vi "getTemperatures (SubVI).vi"(8 "error in (no error)":errorcluster, 10 "file path (dialog if empty)":path, 11 "Application in":refnum<vi>) -> (0 "error out":errorcluster, 1 "Application ref out":refnum<vi>, 2 "TCryo":dbl, 3 "TSTM":dbl)   [LabVIEW 2014]
uses:
  <vilib>/Utility/file.llb/Write To Spreadsheet File (DBL).vi
  <vilib>/Utility/file.llb/Read From Spreadsheet File (DBL).vi
  <userlib>/Nanonis Prog Interface V5/Nanonis Prog Interface.lvlib
  <vilib>/gmath/NI_Gmath.lvlib
panel:
  out "error":i32
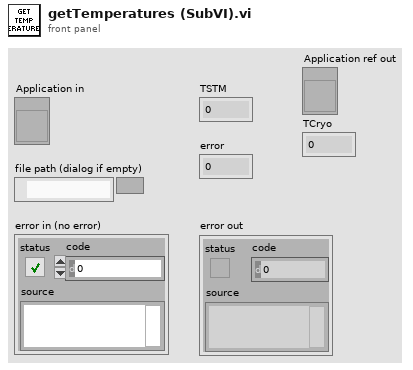
[diagram p1: front panel]
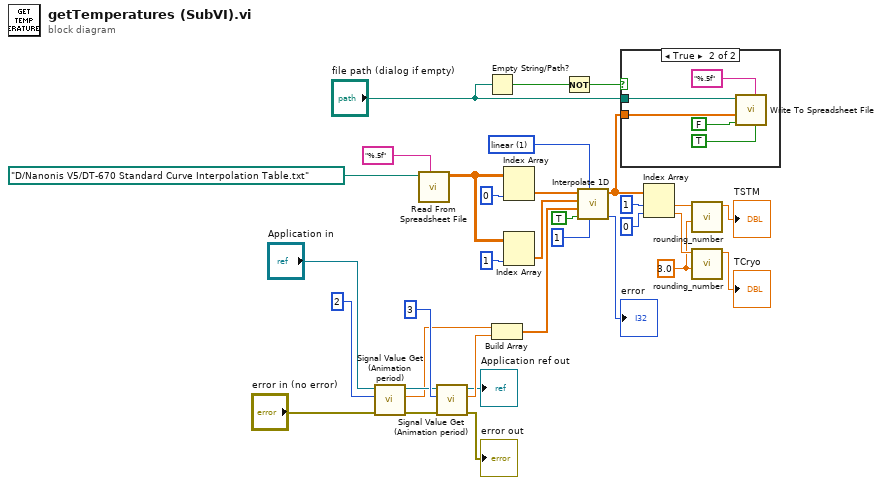
[diagram p0: block diagram]
diagram:
  w1 = 3.0 ("decimal Places")
  w21 = 1 items=["nearest", "linear", "spline", "cubic Hermite", "Lagrange"] ("method")
  n1 = call <userlib>:"Signal Value Get (Animation period).vi"("error in (no error)"="error in (no error)", "Signal index (0-47)"=i8 2, "Application ref in"="Application in") -> ("error out"=w30:errorcluster, "Signal value"=w24:sgl, "Application ref out"=w31:refnum<vi>)  [unwired: 5 in]
  n2 = call-poly <vilib>:"Read From Spreadsheet File.vi"("format (%.3f)"="%.5f", "file path (dialog if empty)"=path "D:/Nanonis V5/DT-670 Standard Curve Interpolation Table.txt") -> ("all rows"=w18:dbl[][])  [unwired: 5 in, 4 out]
  n3 = call <userlib>:"Signal Value Get (Animation period).vi"("error in (no error)"=w30, "Signal index (0-47)"=i8 3, "Application ref in"=w31) -> ("error out"=→"error out":errorcluster, "Signal value"=w32:sgl, "Application ref out"=→"Application ref out":refnum<vi>)  [unwired: 5 in]
  n4 = Empty String/Path?(string/path="file path (dialog if empty)") -> (empty?=w6:bool)
  n5 = Build Array(w24, w32) -> (w25:sgl[])
  n6 = Index Array(array=w18, index (col)=0 ("index")) -> (element=w20:dbl[])  [unwired: 1 in]
  n7 = Index Array(array=w18, index (col)=1 ("index")) -> (element=w17:dbl[])  [unwired: 1 in]
  n8 = Not(x=w6) -> (.not. x?=w8:bool)
  n9 = call <vilib>:"Interpolate 1D.vi"("ntimes"=1, "method"=w21, "X is monotonic"=TRUE, "xi"=w25, "X"=w17, "Y"=w20) -> ("error"=→"error":i32, "yi"=w28:dbl[])  [unwired: 3 in, 1 out]
  n10 = case shown="True" w8 {
    tunnel: w28 -> [_ w37]
    tunnel: "file path (dialog if empty)" -> [_ w34]
    frame False {
    }
    frame True {
      n11 = call-poly <vilib>:"Write To Spreadsheet File.vi"("transpose? (no:F)"=TRUE, "format (%.3f)"="%.5f", "append to file? (new file:F)"=FALSE, "1D data"=w37, "file path (dialog if empty)"=w34) -> ()  [unwired: 3 in, 1 out]
    }
  }
  n12 = Index Array(array=w28, index #1=1 ("index"), index #2=0 ("index")) -> (element #1=w5:dbl, element #2=w3:dbl)
  n13 = call "rounding_number.vi"("decimal Places"=w1, "Numeric"=w5) -> ("rounded number"=→"TSTM":dbl)  [unwired: 9 in]
  n14 = call "rounding_number.vi"("decimal Places"=w1, "Numeric"=w3) -> ("rounded number"=→"TCryo":dbl)  [unwired: 9 in]
